vi "Init Data Logger.vi"(0 "Log File Path":path, 5 "Module":string, 7 "Sevice":string, 11 "error in":errorcluster) -> (4 "Log File Ref. Out":refnum<file>, 6 "Cancelled":bool, 15 "error out":errorcluster)   [LabVIEW 2024, in "dataLogger.lvlib"]
doc: "<B>Create Log</B> API. Input the log file path and file name to initialize and create a log file."
uses:
  dataLogger.lvlib
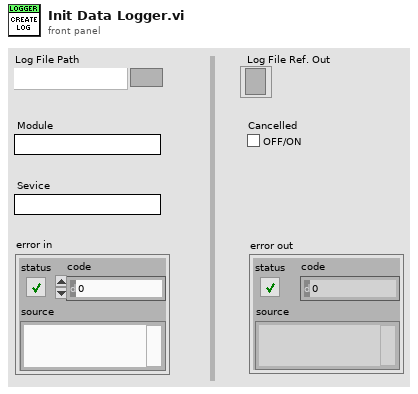
[diagram p1: front panel]
types:
  T1 = enum16{"open", "replace", "create", "open or create", "replace or create", "replace or create with confirmation"}
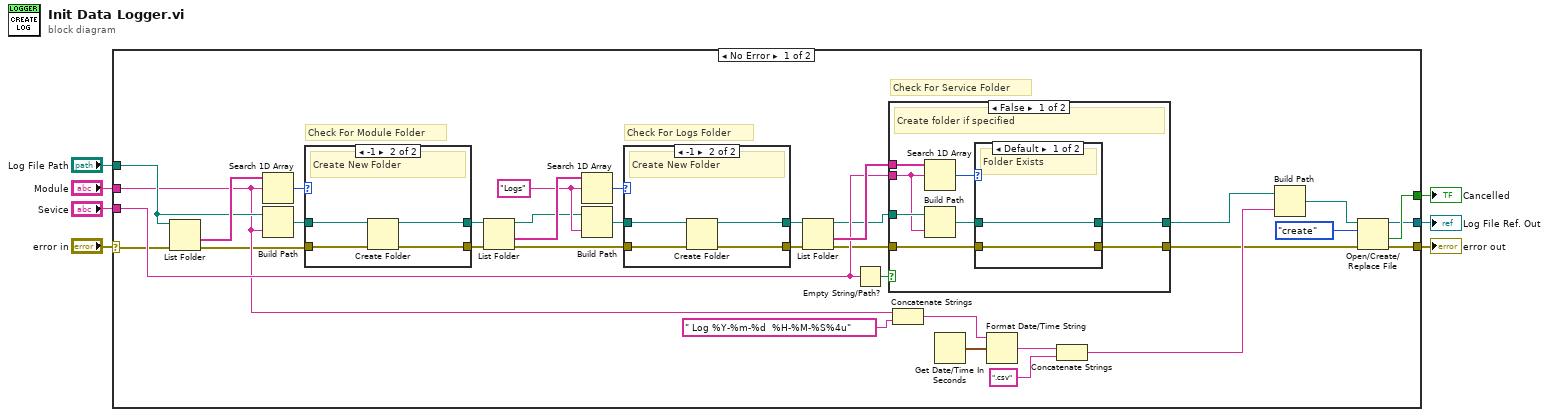
[diagram p0: block diagram]
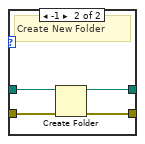
[diagram p3: hidden frame]
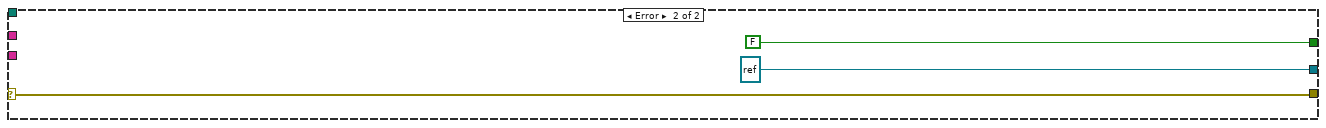
[diagram p6: hidden frame]
diagram:
  n1 = case shown="No Error" "error in" {
    selector: "error in" -> [w23 w73]
    tunnel: "Log File Path" -> [w29 _]
    tunnel: "Module" -> [w27 _]
    tunnel: "Sevice" -> [w28 _]
    tunnel: [w18 w73] -> w4
    tunnel: [w24 FALSE ("cancelled")] -> w3
    tunnel: [w19 refnum<file> refnum ("refnum out")] -> w2
    frame No Error {
      w10 = "Logs" ("element")
      # "Check For Logs Folder"
      # "Check For Service Folder"
      # "Check For Module Folder"
      n2 = List Folder(path=w29, error in=w23) -> (folder names=w40:string[], error out=w22:errorcluster)  [unwired: 2 in, 2 out]
      n3 = Search 1D Array(1D array=w40, element=w27) -> (index of element=w39:i32)  [unwired: 1 in]
      n4 = Build Path(base path=w29, name or relative path=w27) -> (appended path=w41:path)
      n5 = case shown="-1" w39 {
        tunnel: w41 -> [w66 w70]
        tunnel: [w66 w69] -> w12
        tunnel: [w65 w68] -> w14
        tunnel: w22 -> [w65 w67]
        frame Default {
          # "Folder Exists"
        }
        frame -1 {
          # "Create New Folder"
          n6 = Create Folder(path (use dialog)=w70, error in=w67) -> (created path=w69:path, error out=w68:errorcluster)  [unwired: 1 in, 1 out]
        }
      }
      n7 = List Folder(path=w12, error in=w14) -> (path out=w9:path, folder names=w11:string[], error out=w13:errorcluster)  [unwired: 2 in, 1 out]
      n8 = Search 1D Array(1D array=w11, element=w10) -> (index of element=w17:i32)  [unwired: 1 in]
      n9 = Build Path(base path=w9, name or relative path=w10) -> (appended path=w16:path)
      n10 = case shown="-1" w17 {
        tunnel: w16 -> [w44 w48]
        tunnel: [w44 w47] -> w8
        tunnel: [w43 w46] -> w15
        tunnel: w13 -> [w43 w45]
        frame Default {
          # "Folder Exists"
        }
        frame -1 {
          # "Create New Folder"
          n11 = Create Folder(path (use dialog)=w48, error in=w45) -> (created path=w47:path, error out=w46:errorcluster)  [unwired: 1 in, 1 out]
        }
      }
      n12 = List Folder(path=w8, error in=w15) -> (path out=w20:path, folder names=w38:string[], error out=w21:errorcluster)  [unwired: 2 in, 1 out]
      n13 = Empty String/Path?(string/path=w28) -> (empty?=w31:bool)
      n14 = case shown="False" w31 {
        tunnel: w38 -> [w56 _]
        tunnel: w20 -> [w54 w64]
        tunnel: w28 -> [w53 _]
        tunnel: [w51 w64] -> w34
        tunnel: [w50 w63] -> w30
        tunnel: w21 -> [w49 w63]
        frame False {
          # "Create folder if specified"
          n15 = Search 1D Array(1D array=w56, element=w53) -> (index of element=w55:i32)  [unwired: 1 in]
          n16 = Build Path(base path=w54, name or relative path=w53) -> (appended path=w52:path)
          n17 = case shown="Default" w55 {
            tunnel: w52 -> [w58 w62]
            tunnel: [w58 w61] -> w51
            tunnel: [w57 w60] -> w50
            tunnel: w49 -> [w57 w59]
            frame Default {
              # "Folder Exists"
            }
            frame -1 {
              # "Create New Folder"
              n18 = Create Folder(path (use dialog)=w62, error in=w59) -> (created path=w61:path, error out=w60:errorcluster)  [unwired: 1 in, 1 out]
            }
          }
        }
        frame True {
          # "Don't create subfolder"
        }
      }
      n19 = Concatenate Strings(w27, " Log %Y-%m-%d  %H-%M-%S%4u" ("time format string (%c)")) -> (w25:string)
      n20 = Get Date/Time In Seconds() -> (seconds since 1Jan1904=w37:timestamp)
      n21 = Format Date/Time String(time format string (%c)=w25, seconds (now)=w37) -> (date/time string=w36:string)  [unwired: 1 in]
      n22 = Concatenate Strings(w36, ".csv" ("string")) -> (w33:string)
      n23 = Build Path(base path=w34, name or relative path=w33) -> (appended path=w32:path)
      n24 = Open/Create/Replace File(file path (use dialog)=w32, error in=w30, operation (0:open)=T1."create") -> (refnum out=w19:refnum<file>, cancelled=w24:bool, error out=w18:errorcluster)  [unwired: 3 in]
    }
    frame Error {
    }
  }
  "error out" <- w4
  "Cancelled" <- w3
  "Log File Ref. Out" <- w2
